vi "Check Expiration.vi"(0 "Charact Result Accessor in":refnum<class "Result Accessor.lvclass">, 11 "error in":errorcluster) -> (4 "Charact Result Accessor out":refnum<class "Result Accessor.lvclass">, 6 "Expired?":bool, 15 "error out":errorcluster)   [LabVIEW 2023, in "RFCalAndFixtureCharact.Common.lvlib" / "Result Accessor.lvclass"]
uses:
  Result Accessor.lvclass
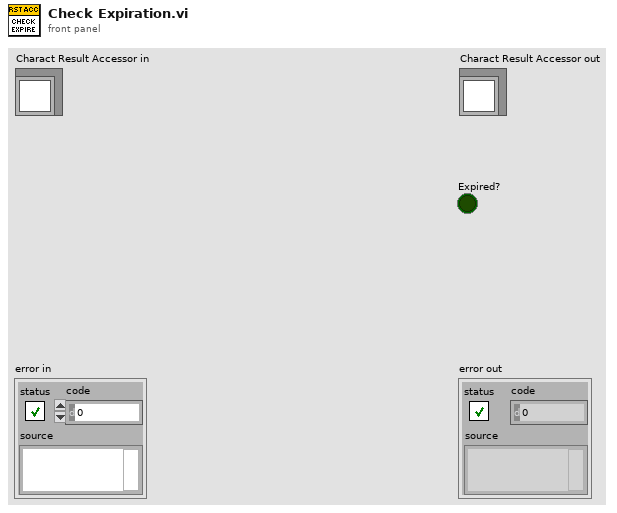
[diagram p1: front panel]
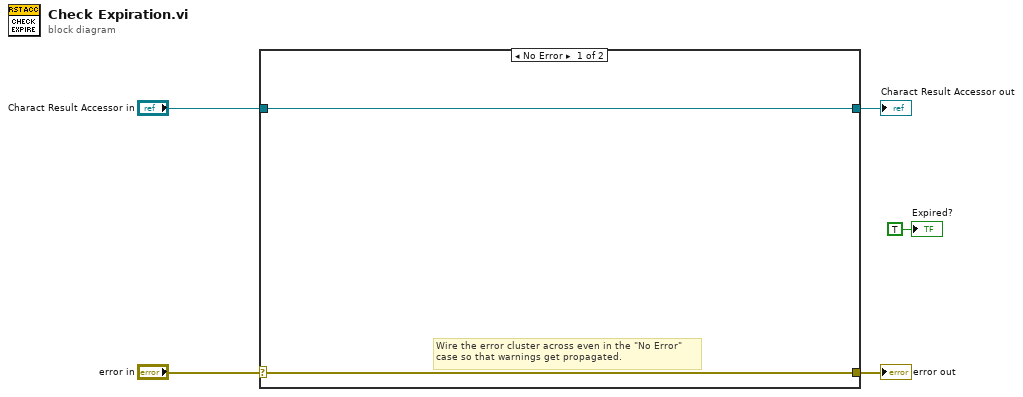
[diagram p0: block diagram]
diagram:
  n1 = case shown="No Error" "error in" {
    selector: "error in" -> [w6 w9]
    tunnel: [w6 w9] -> w4
    tunnel: [w7 w8] -> w2
    tunnel: "Charact Result Accessor in" -> [w7 w8]
    frame No Error {
      # "Wire the error cluster across even in the \"No Error\"\ncase so that warnings get propagated."
    }
    frame Error {
    }
  }
  "error out" <- w4
  "Charact Result Accessor out" <- w2
  "Expired?" <- TRUE ("Expired?")
